vi "HEWH Draw Routing Start.vi"(11 "Start Draw Routine":bool) -> (3 "Start Draw Routine Output":bool)   [LabVIEW 2019]
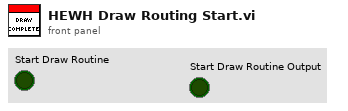
[diagram p1: front panel]
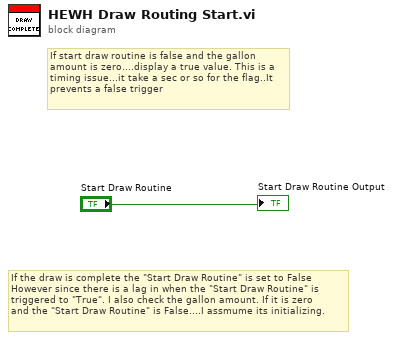
[diagram p0: block diagram]
diagram:
  # "If the draw is complete the \"Start Draw Routine\" is set to False\nHowever since there is a lag in when the \"Start Draw Routine\" is \ntriggered to \"True\". I also check the gallon amount. If it is zero\nand the \"Start Draw Routine\" is False....I assmume its initializing."
  # "If start draw routine is false and the gallon\namount is zero....display a true value. This is a\ntiming issue...it take a sec or so for the flag..It\nprevents a false trigger"
  "Start Draw Routine Output" <- "Start Draw Routine"
